vi "Front.vi"() -> ()   [LabVIEW 2021]
uses:
  Demo_client/RPC Messages/Communication_ControlStream.ctl
  <vilib>/gRPC/LabVIEW gRPC Library/Shared/grpcId.ctl
  Demo_client/Demo_client.lvlib
  <vilib>/gRPC/LabVIEW gRPC Library/grpc-lvsupport-release.lvlib
panel:
  out "size(s)":i32
  in  "Request Data":T1
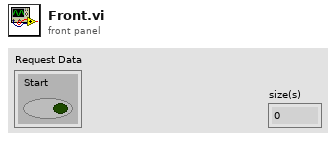
[diagram p1: front panel]
types:
  T1 = typedef "Demo_client.lvlib/Communication_ControlStream.ctl" = cluster{"Start":bool}
  T2 = typedef "grpc-lvsupport-release.lvlib/grpcId.ctl" = u64
  T3 = cluster{"Call Id":T2, "data":i32[], "Start?":bool, "Stream Used?":bool}
  T4 = typedef "Demo_client.lvlib/Communication_StreamData.ctl" = cluster{"data":i32, "Status":bool}
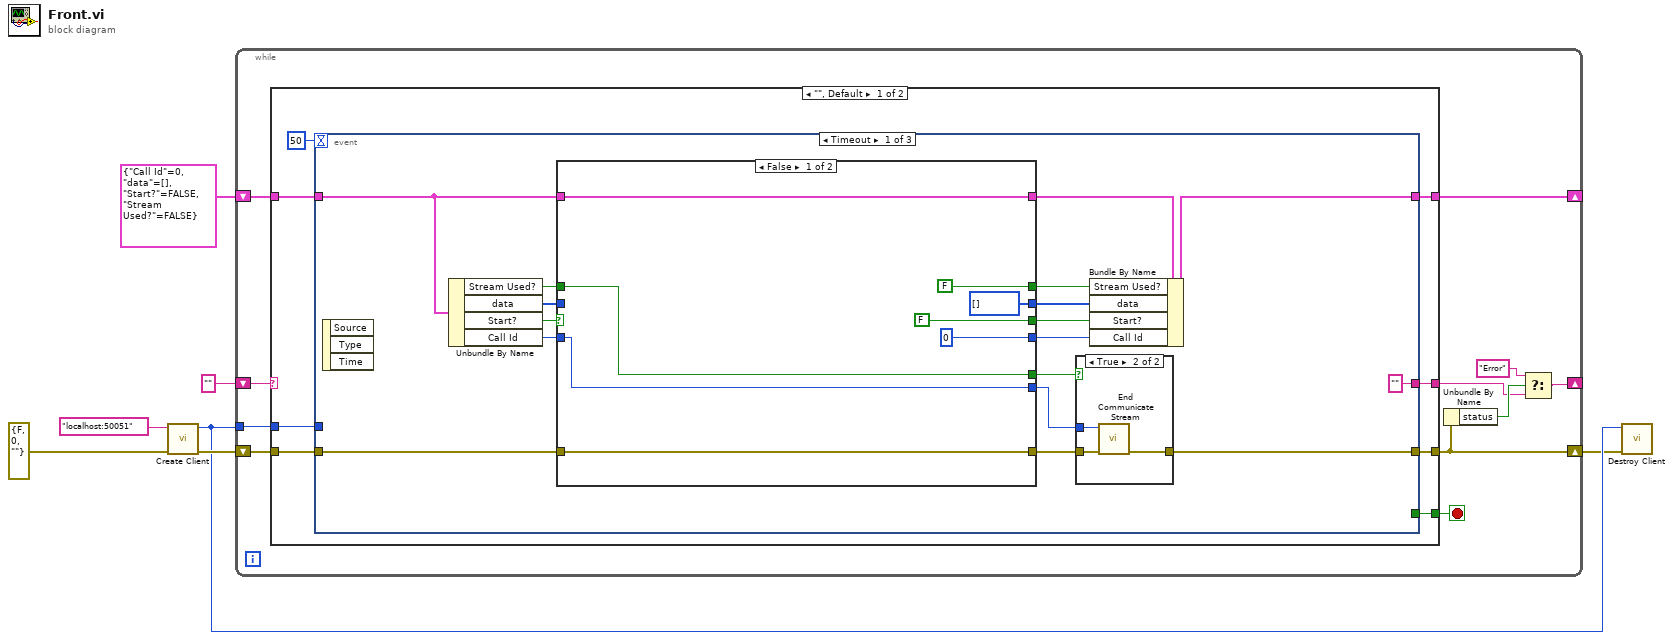
[diagram p0: block diagram]
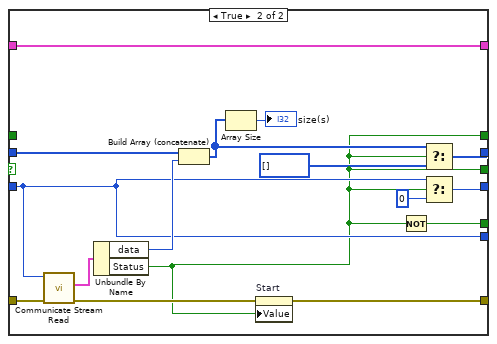
[diagram p3: hidden frame]
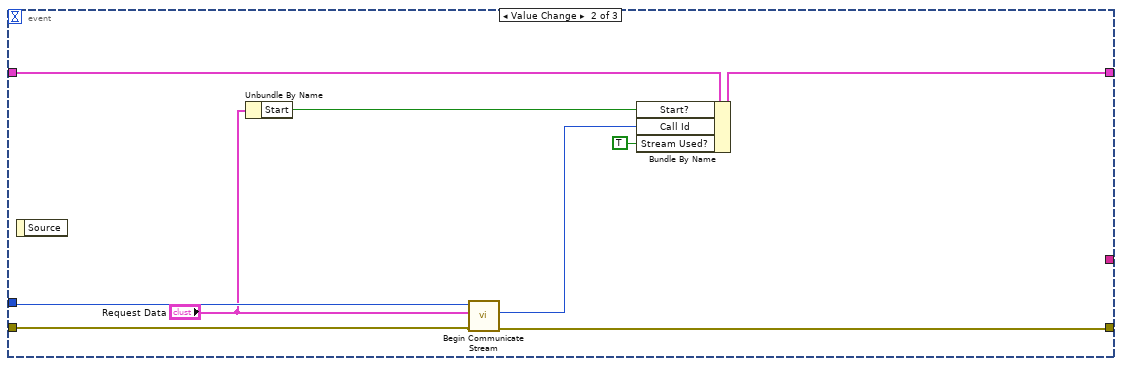
[diagram p4: hidden frame]
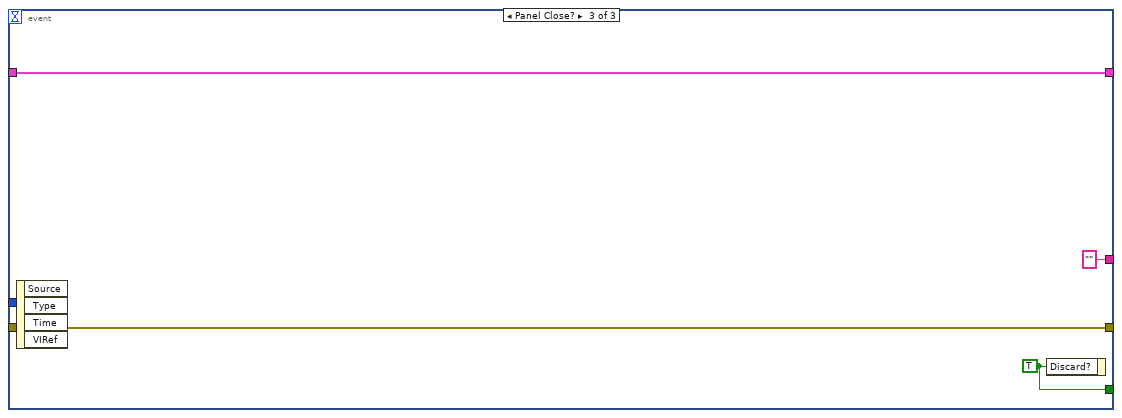
[diagram p5: hidden frame]
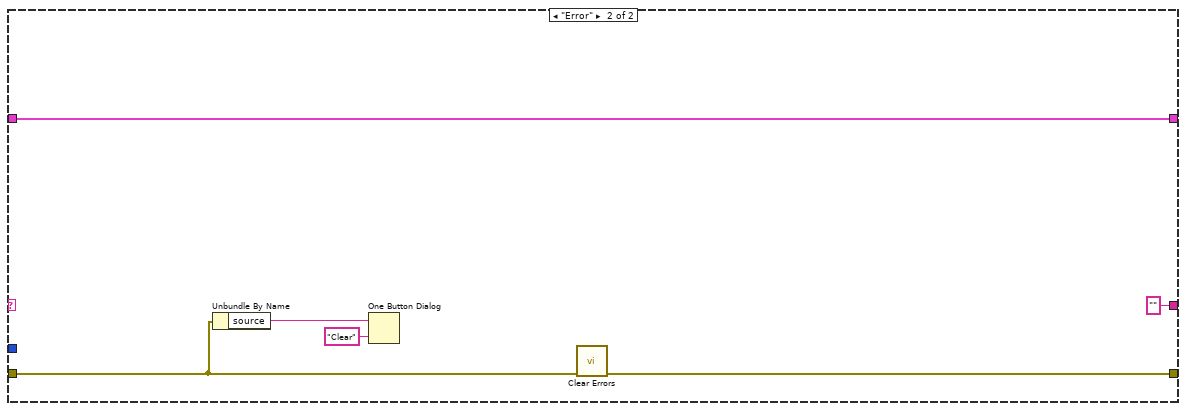
[diagram p6: hidden frame]
diagram:
  n1 = call "Create Client.vi"("error in"=errorcluster {"status"=FALSE, "code"=0, "source"=""} ("error in (no error)"), "address"="localhost:50051") -> ("error out"=w6:errorcluster, "gRPC ID Out"=w3:T2)  [unwired: 8 in]
  n2 = while {
    shift-right: [w14] -> w1
    shift-left: w6 -> [w17]
    tunnel: w3 -> [w16]
    shift-right: [w12] -> _
    shift-left: "" -> [w18]
    shift-right: [w8] -> _
    shift-left: T3 {"Call Id"=0, "data"=[], "Start?"=FALSE, "Stream Used?"=FALSE} -> [w9]
    stop <- w15 stop-if-true
    n3 = case shown="\"\", Default" w18 {
      tunnel: w17 -> [w26 w89]
      tunnel: [w25 w90] -> w14
      tunnel: w16 -> [w24 _]
      tunnel: [w23 ""] -> w11
      tunnel: [w22 _] -> w15
      tunnel: w9 -> [w20 w85]
      tunnel: [w19 w85] -> w8
      frame "", Default {
        n4 = event shown="[0] Timeout" {
          selector: _ -> [_ _ _]
          dyn-events: _ -> [_ _ _]
          timeout: 50 -> [_ _ _]
          tunnel: w26 -> [w42 w79 w84]
          tunnel: [w31 w74 w84] -> w25
          tunnel: w24 -> [_ w80 _]
          tunnel: ["" _ ""] -> w23
          tunnel: [_ _ w82] -> w22
          tunnel: w20 -> [w40 w77 w81]
          tunnel: [w36 w78 w81] -> w19
          event Timeout {
            n5 = event-data() -> ()  [unwired: 1 in, 3 out]
            n6 = Unbundle By Name(w40) -> ("Stream Used?"=w33:bool, "data"=w37:i32[], "Start?"=w39:bool, "Call Id"=w38:T2)
            n7 = case shown="False" w39 {
              tunnel: [w53 w64] -> w30
              tunnel: w42 -> [w53 w70]
              tunnel: w40 -> [w55 w71]
              tunnel: [w55 w71] -> w41
              tunnel: w38 -> [w50 w62]
              tunnel: w37 -> [_ w68]
              tunnel: [i32[] [] ("f") w59] -> w35
              tunnel: [FALSE w56] -> w34
              tunnel: w33 -> [w51 _]
              tunnel: [FALSE ("Stream Used?") w56] -> w32
              tunnel: [w51 w60] -> w27
              tunnel: [w50 w62] -> w29
              tunnel: [T2 0 ("Call Id") w63] -> w28
              frame False {
              }
              frame True {
                n8 = call "Communicate Stream Read.vi"("error in"=w70, "Call ID in"=w62) -> ("error out"=w65:errorcluster, "Response Data"=w69:T4)  [unwired: 6 in, 2 out]
                n9 = Unbundle By Name(w69) -> ("data"=w67:i32, "Status"=w56:bool)
                n10 = Build Array (concatenate)(w68, w67) -> (w58:i32[])
                n11 = Array Size(array=w58) -> (size(s)=→"size(s)":i32)
                n12 = property on="Start" class="Bool (strict)"(error in=w65, "Value"=w56) -> (error out=w64:errorcluster)  [unwired: 1 in, 1 out]
                n13 = Not(x=w56) -> (.not. x?=w60:bool)
                n14 = Select(t=w58, s=w56, f=i32[] []) -> (s? t:f=w59:i32[])
                n15 = Select(t=w62, s=w56, f=T2 0) -> (s? t:f=w63:T2)
              }
            }
            n16 = case shown="True" w27 {
              tunnel: [w44 w47] -> w31
              tunnel: w30 -> [w44 w46]
              tunnel: w29 -> [_ w45]
              frame False {
              }
              frame True {
                n17 = call "End Communicate Stream.vi"("error in"=w46, "Call ID in"=w45) -> ("error out"=w47:errorcluster)  [unwired: 8 in, 1 out]
              }
            }
            n18 = Bundle By Name(cluster=w41, "Stream Used?"=w32, "data"=w35, "Start?"=w34, "Call Id"=w28) -> (w36:T3)
          }
          event Value Change {
            n19 = event-data() -> ()  [unwired: 1 in, 1 out]
            n20 = Unbundle By Name("Request Data") -> ("Start"=w75:bool)
            n21 = call "Begin Communicate Stream.vi"("error in"=w79, "Request Data"="Request Data", "gRPC ID"=w80) -> ("error out"=w74:errorcluster, "Call Id Out"=w76:T2)  [unwired: 6 in, 1 out]
            n22 = Bundle By Name(cluster=w77, "Start?"=w75, "Call Id"=w76, "Stream Used?"=TRUE) -> (w78:T3)
          }
          event Panel Close? {
            w82 = TRUE ("Discard?")
            n23 = event-data() -> ()  [unwired: 1 in, 4 out]
            n24 = event-data("Discard?"=w82) -> ()  [unwired: 1 in, 1 out]
          }
        }
      }
      frame "Error" {
        n25 = Unbundle By Name(w89) -> ("source"=w87:string)
        n26 = One Button Dialog(message=w87, button name ("OK")="Clear") -> ()  [unwired: 1 out]
        n27 = call <vilib>:"Clear Errors.vi"("error in (no error)"=w89) -> ("error out"=w90:errorcluster)  [unwired: 5 in, 1 out]
      }
    }
    n28 = Unbundle By Name(w14) -> ("status"=w13:bool)
    n29 = Select(t="Error", s=w13, f=w11) -> (s? t:f=w12:string)
  }
  n30 = call "Destroy Client.vi"("error in"=w1, "gRPC ID"=w3) -> ()  [unwired: 9 in, 1 out]
